vi "Target Converter.vi"(11 "Array":dbl[](array[numeric])) -> (3 "Target type":T1)   [LabVIEW 2013]
uses:
  Target Type.ctl
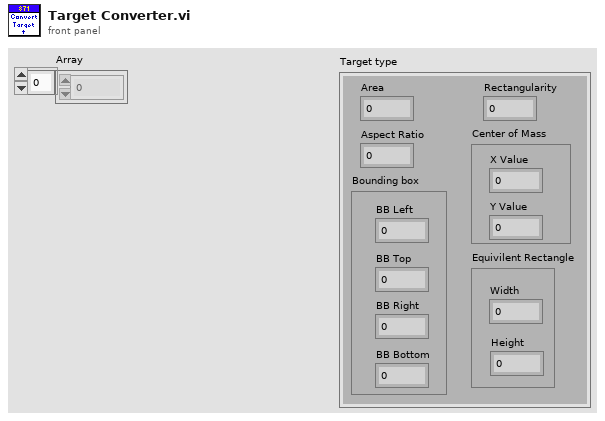
[diagram p1: front panel]
types:
  T1 = typedef "Target Type.ctl" = cluster{"Area":dbl, "Bounding box":cluster{"BB Left":dbl, "BB Top":dbl, "BB Right":dbl, "BB Bottom":dbl}, "Center of Mass":cluster{"X Value":dbl, "Y Value":dbl}, "Equivilent Rectangle":cluster{"Width":dbl, "Height":dbl}, "Aspect Ratio":dbl, "Rectangularity":dbl}
  T2 = cluster{"Numeric":dbl, "Numeric":dbl, "Numeric":dbl, "Numeric":dbl}
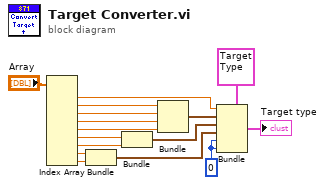
[diagram p0: block diagram]
diagram:
  w1 = 0
  n1 = Index Array(array="Array") -> (element #1=w13:dbl, element #2=w11:dbl, element #3=w10:dbl, element #4=w9:dbl, element #5=w8:dbl, element #6=w7:dbl, element #7=w6:dbl, element #8=w4:dbl, element #9=w3:dbl)  [unwired: 9 in]
  n2 = Bundle("Numeric"=w4, "Numeric"=w3) -> (w2:cluster{"Numeric":dbl, "Numeric":dbl})  [unwired: 1 in]
  n3 = Bundle("Numeric"=w7, "Numeric"=w6) -> (w5:cluster{"Numeric":dbl, "Numeric":dbl})  [unwired: 1 in]
  n4 = Bundle("Numeric"=w11, "Numeric"=w10, "Numeric"=w9, "Numeric"=w8) -> (w12:T2)  [unwired: 1 in]
  n5 = Bundle(cluster=T1 {"Area"=0.0, "Bounding box"={"BB Left"=0.0, "BB Top"=0.0, "BB Right"=0.0, "BB Bottom"=0.0}, "Center of Mass"={"X Value"=0.0, "Y Value"=0.0}, "Equivilent Rectangle"={"Width"=0.0, "Height"=0.0}, "Aspect Ratio"=0.0, "Rectangularity"=0.0} ("Target type"), "Area"=w13, "Bounding box"=w12, "Center of Mass"=w5, "Equivilent Rectangle"=w2, "Aspect Ratio"=w1, "Rectangularity"=w1) -> (→"Target type":T1)
